vi "Get Worksheet.Name.vi"(8 "error in (no error)":errorcluster, 11 "worksheet in":refnum<class "worksheet.lvclass">) -> (0 "error out":errorcluster, 2 "String":string, 3 "worksheet out":refnum<class "worksheet.lvclass">)   [LabVIEW 2017, in "Excel_Specific.lvlib" / "worksheet.lvclass"]
uses:
  worksheet.lvclass
  worksheet.lvclass/worksheet.ctl
  C:/Users/Neo/Desktop/Dev_Tools_BR/LabVIEW_NPOI/src/lib/NPOI 2.1.1/NPOI.dll
  lib/NPOI 2.1.1/NPOI.dll
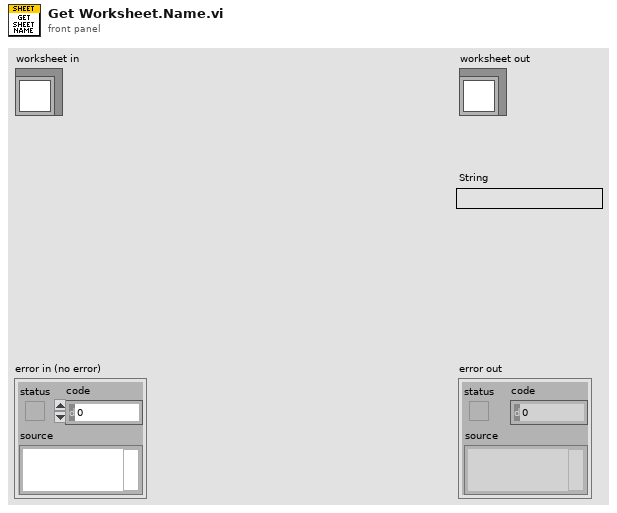
[diagram p1: front panel]
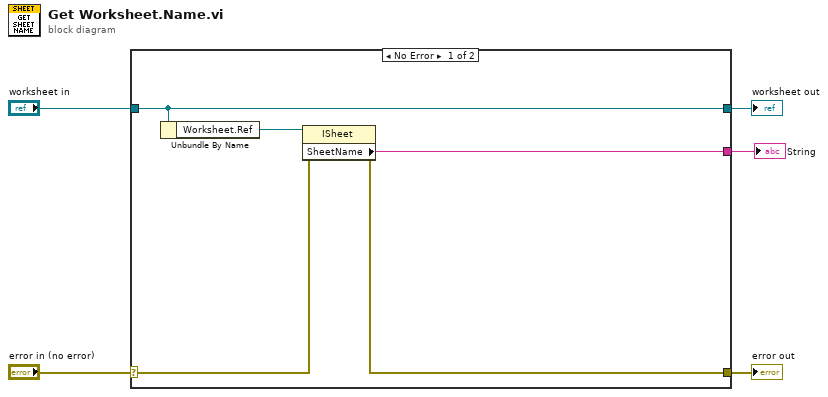
[diagram p0: block diagram]
diagram:
  n1 = case shown="No Error" "error in (no error)" {
    selector: "error in (no error)" -> [w8 w12]
    tunnel: [w7 w12] -> w4
    tunnel: [w10 w11] -> w2
    tunnel: "worksheet in" -> [w10 w11]
    tunnel: [w6 _] -> w1
    frame No Error {
      n2 = Unbundle By Name(w10) -> ("Worksheet.Ref"=w9:refnum<k24>)
      n3 = property class="ISheet"(reference=w9, error in=w8) -> (error out=w7:errorcluster, "SheetName"=w6:string)  [unwired: 1 out]
    }
    frame Error {
    }
  }
  "error out" <- w4
  "worksheet out" <- w2
  "String" <- w1
